vi "Compute Maximum Power of 2.vi"(11 "Total Global Memory (Bytes)":i64) -> (3 "Max N":i32)   [LabVIEW 2020, in "Get GPU Device Information.lvlib"]
uses:
  Get GPU Device Information.lvlib
  <vilib>/addons/lvgpu/utility/Byte Size of CSG.vi
  <vilib>/addons/lvgpu/utility/Byte Size of SGL.vi
  <vilib>/addons/lvgpu/lvgpusdk.lvlib
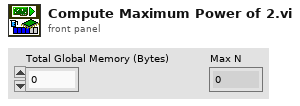
[diagram p1: front panel]
types:
  T1 = typedef "lvgpusdk.lvlib/size_t.ctl" = i64
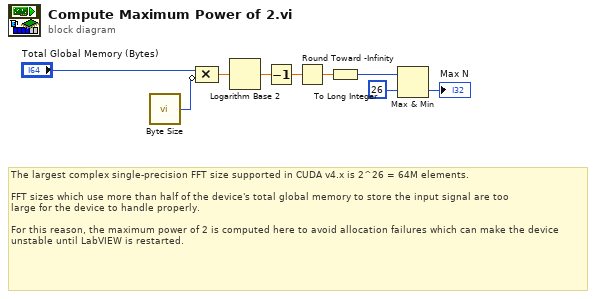
[diagram p0: block diagram]
diagram:
  # "The largest complex single-precision FFT size supported in CUDA v4.x is 2^26 = 64M elements.\n\nFFT sizes which use more than half of the device's total global memory to store the input signal are too \nlarge for the device to handle properly.\n\nFor this reason, the maximum power of 2 is computed here to avoid allocation failures which can make the device unstable until LabVIEW is restarted."
  n1 = call-poly <vilib>:"Byte Size.vi"() -> ("size in bytes"=w2:T1)  [unwired: 1 in]
  n2 = Compound Arithmetic op=MULTIPLY("Total Global Memory (Bytes)", invert w2) -> (w3:dbl)
  n3 = Logarithm Base 2(1:w3) -> (0:w4:dbl)
  n4 = Decrement(x=w4) -> (x-1=w5:dbl)
  n5 = Round Toward -Infinity(1:w5) -> (0:w6:dbl)
  n6 = To Long Integer(number=w6) -> (32bit integer=w7:i32)
  n7 = Max & Min(x=w7, y=26) -> (min(x,y)=→"Max N":i32)  [unwired: 1 out]
